vi "WaitBallTrajSkill.vi"(6 "passer tactic":T1=enum."PenaltyAttacker", 7 "firstCall":bool, 8 "error in (no error)":errorcluster, 9 "Robot":refnum<class "Robot.lvclass">, 10 "Game":refnum<class "Game.lvclass">, 11 "WaitBallTrajSkill in":refnum<class "WaitBallTrajSkill.lvclass">) -> (0 "error out":errorcluster, 2 "robot out":refnum<class "Robot.lvclass">, 3 "WaitBallTrajSkill out":refnum<class "WaitBallTrajSkill.lvclass">)   [LabVIEW 2024, in "WaitBallTrajSkill.lvclass"]
uses:
  WaitBallTrajSkill.lvclass
  Game_class/Game.lvclass
  Robot_class/Robot.lvclass
  C:/Users/moise/Documents/GitHub/SSL_AI/Object_class/Object.lvclass
  Robot_class/tactics.ctl
  Robot_class/robotKickToStates.ctl
  Robot_class/roles.ctl
  Robot_class/Robot.lvclass/Robot.ctl
  Object_class/Object.lvclass/Object.ctl
  Game_class/Game.lvclass/Game.ctl
  Parameters_class/Parameters.lvclass/Parameters.ctl
  Team_class/Team.lvclass/Team.ctl
  Ball_class/Ball.lvclass/Ball.ctl
  Field_class/Field.lvclass/Field.ctl
  Parameters_class/Read KickForce.vi
  Game_class/Read Parameters.lvclass.vi
  Game_class/Read BallRef.vi
  Game_class/Read Utilities.lvclass.vi
  Game_class/Read FieldRef.vi
  Game_class/Read NewParameters.vi
  Game_class/Read KeeperTeam.vi
  Game_class/Read OffensiveTeam.vi
  Team_class/Read RobotRef.vi
  Team_class/Read KeeperPlay.vi
  Field_class/Read ourGoalPosition.vi
  Field_class/Read enemyGoalPosition.vi
  Object_class/Read position(x,y).vi
  Ball_class/Read velocityNorm.vi
  Parameters_class/Read BallVelToAbortPass.vi
  Parameters_class/Read AttakingOurselves.vi
  Robot_class/Read Zone.vi
  Robot_class/Write robotKickState.vi
  Robot_class/Write dest_x.vi
  Robot_class/Write dest_y.vi
  Robot_class/Write dest_orientation.vi
  Robot_class/Write dribble.vi
  Robot_class/Write kick_x.vi
  Robot_class/Write keepDest.vi
  <vilib>/Analysis/_algsub.llb/Vector Norm.vi
  <vilib>/Analysis/_algsub.llb/Real Vector Norm.vi
  Ally_class/Ally.lvclass
  C:/Users/moise/Documents/GitHub/SSL_AI/Team_class/Team.lvclass
  Ball_class/Ball.lvclass
  Parameters_class/Parameters.lvclass
  Utilities_class/Utilities.lvclass
  Field_class/Field.lvclass
  Zone_class/Zone.lvclass
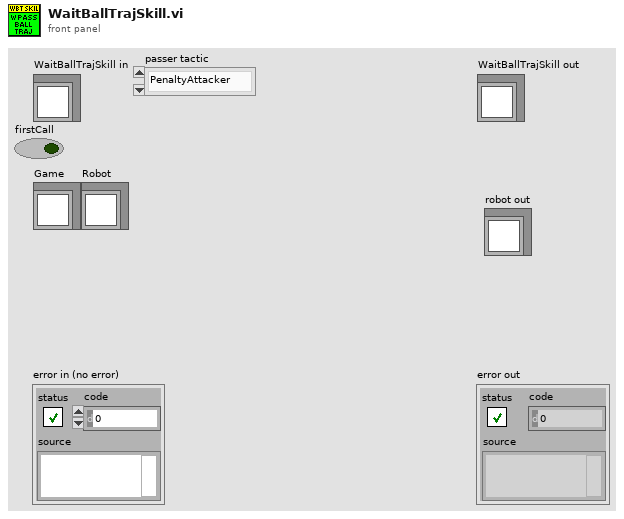
[diagram p1: front panel]
types:
  T1 = typedef "tactics.ctl" = enum16{"GoToBallPlacementPosition", "PlaceBall", "GoToBallPlacement", "5Robots", "BallPlacementEnemy", "ReceivePassInFuturePoint", "Roller", "PrepareRollToPassRollerGoTo", "PrepareRollToPassReceiverGoTo", "WaitRoll", "PositionToRoll", "PenaltyAttacker", "PassObserver", "PenaltyDefense", "TableReceiverTactic", "Test", "DefendGoal", "Marker", "FollowAttacker", "DefendArea", "Shoot", "AttackerAimGoal", "AttackerBallOutOfField", "AttackerBlock", "AttackerStop", "Duelist", "Halt", "ZigZag", "GoTo", "Timeout", "KickToBestRobot", "KickToPassReceiver", "PositionToReceivePass", "WaitPass", "GoToTarget"}
  T2 = typedef "robotKickToStates.ctl" = enum16{"shootFromDirect", "avoidCollideBall", "goToBackBall", "none", "walk", "turn", "turnAntiClockWise", "turnClockwise", "oldKickToShoot", "oldKickToGoToBackBall", "shoot"}
  T3 = typedef "roles.ctl" = enum16{"SimpleBallPlacement", "BallPlacementAllyPasser", "BallPlacementAllyReceiver", "BallPlacementEnemy", "5Robots5th", "PassBestReceiver", "5Robots4th", "5Robots3rd", "5Robots2nd", "5Robots1st", "PassBestRobot", "WaitPass", "ABCThirdKicker", "ABCFirstKicker", "ABCSecondKicker", "Tabler", "TableFinalizer", "PrepareRollToPassRoller", "PrepareRollToPassReceiver", "SimplePassRoll", "SimplePassRollReceiver", "PenaltyDefense", "PreparePassReceiver 2", "PreparePassReceiver 1", "PassObserver", "Timeout", "Goto", "ZigZag", "None", "BallOutOfField", "DefenderArea", "Duelist", "AttackerStop", "FollowAttacker", "KeeperRole", "KickPenalty", "AttackerAimGoal", "AttackerBlock", "Marker", "Halt", "Shoot", "PassKicker", "PassReceiver", "TestRole", "PenaltyAttacker"}
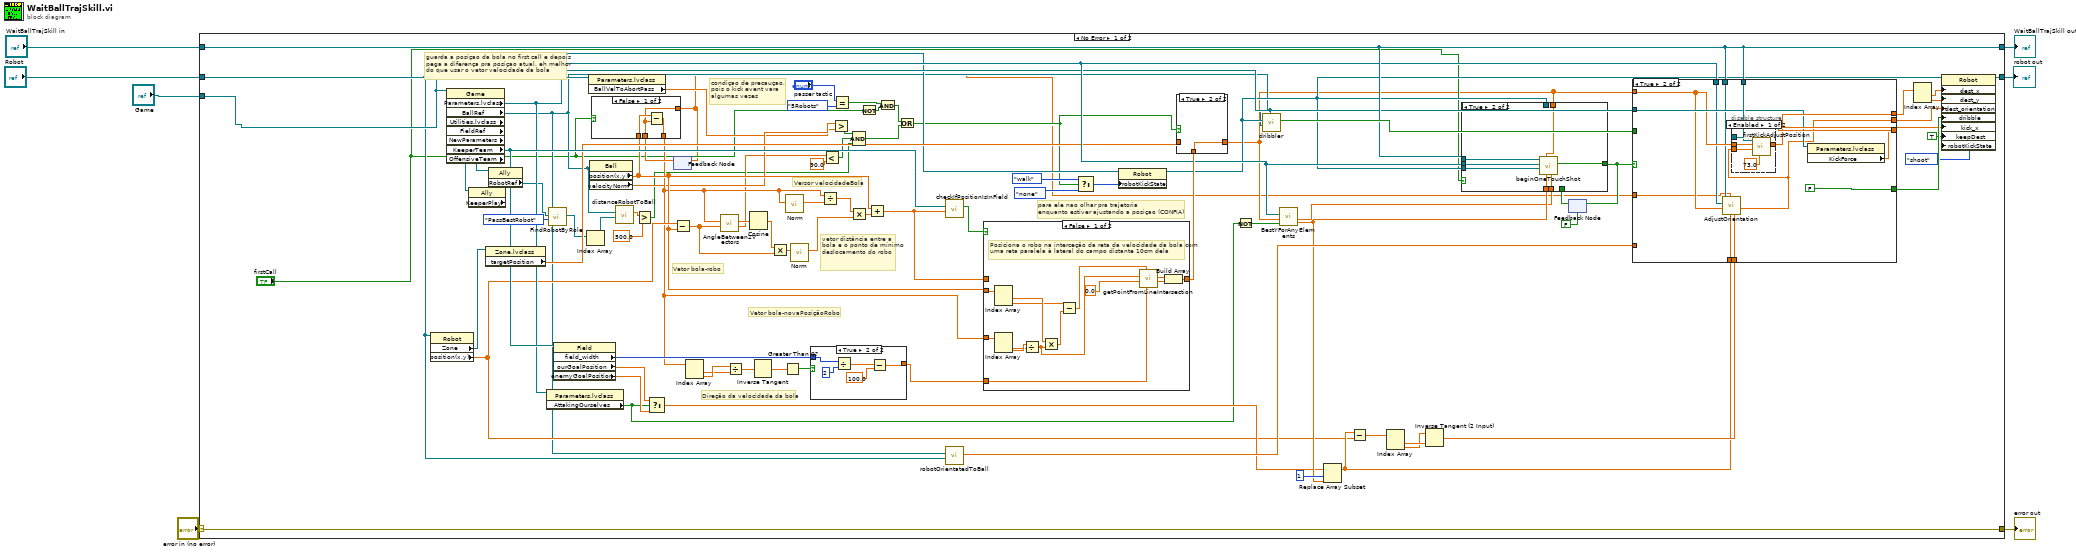
[diagram p0: block diagram]
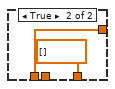
[diagram p2: hidden frame]
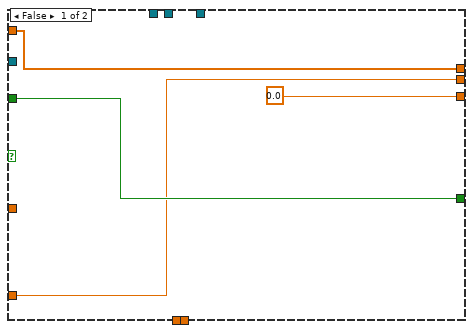
[diagram p4: hidden frame]
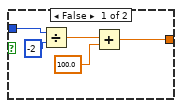
[diagram p7: hidden frame]
diagram:
  n1 = case shown="No Error" "error in (no error)" {
    selector: "error in (no error)" -> [w94 w158]
    tunnel: [w94 w158] -> w6
    tunnel: [w57 w157] -> w4
    tunnel: "WaitBallTrajSkill in" -> [w57 w157]
    tunnel: "Robot" -> [w42 _]
    tunnel: "Game" -> [w56 _]
    tunnel: [w93 _] -> w2
    frame No Error {
      # "guarda a posiçao da bola no first call e depois\npega a diferença pra posiçao atual. eh melhor\ndo que usar o vetor velocidade da bola"
      # "condiçao de precauçao,\npois o kick event vara \nalgumas vezes"
      # "para ele nao olhar pra trajetoria \nenquanto estiver ajustando a posiçao (CONFIA)"
      # "vetor distância entre a bola e o ponto de mínimo deslocamento do robo"
      # "Versor velocidadeBola"
      # "Direção da velocidade da bola"
      # "Vetor bola-novaPosiçãoRobo"
      # "Vetor bola-robo"
      n2 = property class="Robot"(reference=w42) -> ("Zone"=w45:refnum<class "Zone.lvclass">, "position(x,y)"=w46:dbl[])  [unwired: 1 in, 2 out]
      n3 = property class="Game" props=["Parameters.lvclass", "BallRef", "Utilities.lvclass", "FieldRef", "NewParameters", "KeeperTeam", "OffensiveTeam"](reference=w56) -> ("Parameters.lvclass"=w47:refnum<class "Parameters.lvclass">, "BallRef"=w15:refnum<class "Ball.lvclass">, "FieldRef"=w79:refnum<class "Field.lvclass">, "KeeperTeam"=w69:refnum<class "Ally.lvclass">, "OffensiveTeam"=w19:refnum<class "Ally.lvclass">)  [unwired: 1 in, 4 out]
      n4 = property class="Ally" props=["KeeperPlay"](reference=w69) -> ()  [unwired: 1 in, 3 out]
      n5 = property class="Zone.lvclass"(reference=w45) -> ("targetPosition"=w44:dbl[])  [unwired: 1 in, 2 out]
      n6 = property class="Ally"(reference=w19) -> ("RobotRef"=w18:refnum<class "Robot.lvclass">[])  [unwired: 1 in, 2 out]
      n7 = property class="Parameters.lvclass"(reference=w47) -> ("AttakingOurselves"=w51:bool)  [unwired: 1 in, 2 out]
      n8 = call "FindRobotByRole.vi"("role"=roles."PassBestRobot", "RobotRef"=w18) -> ("Robots"=w17:refnum<class "Robot.lvclass">[])  [unwired: 6 in, 3 out]
      n9 = property class="Field"(reference=w79) -> ("field_width"=w70:i32, "ourGoalPosition"=w54:dbl[], "enemyGoalPosition"=w53:dbl[])  [unwired: 1 in, 2 out]
      n10 = Index Array(array=w17) -> (element=w16:refnum<class "Robot.lvclass">)  [unwired: 1 in]
      n11 = property class="Parameters.lvclass"(reference=w47) -> ("BallVelToAbortPass"=w26:dbl)  [unwired: 1 in, 2 out]
      n12 = property class="Ball"(reference=w15) -> ("position(x,y)"=w33:dbl[], "velocityNorm"=w27:dbl)  [unwired: 1 in, 2 out]
      n13 = call "distanceRobotToBall.vi"("Robot"=w16, "Ball"=w15) -> ("Distance Robot To Ball"=w14:dbl)  [unwired: 7 in, 2 out]
      n14 = Greater?(x=w14, y=500.0) -> (0:w12:bool)
      n15 = Select(t=w54, s=w51, f=w53) -> (s? t:f=w52:dbl[])
      n16 = feedback #1() -> (w32:dbl[])  [unwired: 1 in]
      n17 = case shown="False" "firstCall" {
        tunnel: w33 -> [w97 w99]
        tunnel: w32 -> [w96 _]
        tunnel: [w96 w99] -> w9
        tunnel: [w95 dbl[] []] -> w30
        frame False {
          n18 = Subtract(x=w97, y=w96) -> (x-y=w95:dbl[])
        }
        frame True {
        }
      }
      n19 = feedback-in #1(w9) -> ()
      n20 = Subtract(x=w46, y=w33) -> (x-y=w43:dbl[])
      n21 = Index Array(array=w30) -> (element #1=w88:dbl, element #2=w89:dbl)  [unwired: 2 in]
      n22 = call "AngleBetween2Vectors.vi"("Array 1"=w43, "Array 2"=w30) -> ("angleInDegrees"=w21:dbl, "angleInRadians(default)"=w48:dbl)  [unwired: 6 in, 2 out]
      n23 = Divide(x=w89, y=w88) -> (x/y=w87:dbl)
      n24 = Cosine(x=w48) -> (cos(x)=w92:dbl)
      n25 = Inverse Tangent(1:w87) -> (0:w62:dbl)
      n26 = Multiply(x=w92, y=w43) -> (x*y=w83:dbl[])
      n27 = Greater Than 0?(x=w62) -> (x > 0?=w86:bool)
      n28 = call "Norm.vi"("2D vector"=w30) -> ("Modulo"=w31:dbl)  [unwired: 8 in, 2 out]
      n29 = call "Norm.vi"("2D vector"=w83) -> ("Modulo"=w80:dbl)  [unwired: 8 in, 2 out]
      n30 = case shown="True" w86 {
        tunnel: [w135 w140] -> w85
        tunnel: w70 -> [w132 w137]
        frame False {
          n31 = Divide(x=w132, y=-2) -> (x/y=w134:dbl)
          n32 = Add(x=w134, y=100.0) -> (x+y=w135:dbl)
        }
        frame True {
          n33 = Divide(x=w137, y=2) -> (x/y=w139:dbl)
          n34 = Subtract(x=w139, y=100.0) -> (x-y=w140:dbl)
        }
      }
      n35 = Divide(x=w30, y=w31) -> (x/y=w81:dbl[])
      n36 = Less?(x=w21, y=90.0) -> (x < y?=w23:bool)
      n37 = Greater?(x=w27, y=w26) -> (0:w25:bool)
      n38 = Equal?(x="passer tactic", y=tactics."5Robots") -> (x = y?=w35:bool)
      n39 = Multiply(x=w81, y=w80) -> (x*y=w82:dbl[])
      n40 = Compound Arithmetic op=AND(w25, w23, w12) -> (w24:bool)
      n41 = Not(x="firstCall") -> (.not. x?=w34:bool)
      n42 = Add(x=w33, y=w82) -> (x+y=w90:dbl[])
      n43 = And(x=w35, y=w34) -> (x .and. y?=w29:bool)
      n44 = Or(x=w29, y=w24) -> (x .or. y?=w28:bool)
      n45 = call "checkIfPositionIsInField.vi"("Position"=w90, "FieldRef"=w79) -> ("Position Is In Field?"=w91:bool)  [unwired: 5 in, 4 out]
      n46 = call "robotOrientatedToBall.vi"("Robot"=w42, "BallRef"=w15) -> ("Orientation"=w74:dbl)  [unwired: 7 in, 2 out]
      n47 = case shown="False" w91 {
        tunnel: w90 -> [_ w156]
        tunnel: [w153 w156] -> w84
        tunnel: w85 -> [w151 _]
        tunnel: w33 -> [w150 _]
        tunnel: w30 -> [w149 _]
        frame False {
          # "Posiciona o robo na interceção da reta da velocidade da bola com uma reta paralela à lateral do campo distante 10cm dela"
          n48 = Index Array(array=w149) -> (element #1=w147:dbl, element #2=w148:dbl)  [unwired: 2 in]
          n49 = Index Array(array=w150) -> (element #1=w146:dbl, element #2=w145:dbl)  [unwired: 2 in]
          n50 = Divide(x=w148, y=w147) -> (x/y=w142:dbl)
          n51 = Multiply(x=w146, y=w142) -> (x*y=w144:dbl)
          n52 = Subtract(x=w145, y=w144) -> (x-y=w143:dbl)
          n53 = call "getPointFromLineIntersection.vi"("b2"=w151, "b1"=w143, "a2"=0.0, "a1"=w142) -> ("y_intersection"=w154:dbl, "x_intersection"=w155:dbl)  [unwired: 4 in, 2 out]
          n54 = Build Array(w155, w154) -> (w153:dbl[])
        }
        frame True {
        }
      }
      n55 = Select(t=robotKickToStates."walk" ("robotKickState"), s=w28, f=robotKickToStates."none" ("robotKickState")) -> (s? t:f=w38:T2)
      n56 = property class="Robot"(reference=w42, "robotKickState"=w38) -> (reference out=w41:refnum<class "Robot.lvclass">)  [unwired: 1 in, 1 out]
      n57 = case shown="True" w28 {
        tunnel: w84 -> [_ w131]
        tunnel: [w130 w131] -> w10
        tunnel: w44 -> [w130 _]
        frame False {
        }
        frame True {
        }
      }
      n58 = Not(x=w51) -> (.not. x?=w50:bool)
      n59 = call "dribbler.vi"("Parameters.lvclass"=w47, "Ball"=w15, "Robot"=w41) -> ("Dribbler?"=w77:bool)  [unwired: 6 in, 2 out]
      n60 = call "BestYForAnyElements.vi"("inimigos"=w50, "Position to be analyzed"=w10, "Game"=w56) -> ("Best y"=w55:dbl, "Gap Coord"=w49:dbl[])  [unwired: 5 in, 2 out]
      n61 = Replace Array Subset(array=w52, new element=w55, index=1) -> (w58:dbl[])
      n62 = Subtract(x=w58, y=w46) -> (x-y=w71:dbl[])
      n63 = Index Array(array=w71) -> (element #1=w73:dbl, element #2=w72:dbl)  [unwired: 2 in]
      n64 = Inverse Tangent (2 Input)(1:w73, 2:w72) -> (0:w59:dbl)
      n65 = feedback #2(FALSE ("Boolean")) -> (w64:bool)
      n66 = case shown="True" "firstCall" {
        tunnel: w57 -> [_ w107]
        tunnel: w56 -> [_ w106]
        tunnel: w41 -> [_ w105]
        tunnel: [w100 w104] -> w65
        tunnel: w64 -> [w100 _]
        tunnel: w41 -> [_ _]
        tunnel: w55 -> [_ w103]
        tunnel: w49 -> [_ w102]
        tunnel: w10 -> [_ w101]
        frame False {
        }
        frame True {
          n67 = call "beginOneTouchShot.vi"("Gap Coord"=w102, "bestY"=w103, "targetPosition"=w101, "Robot"=w105, "Game"=w106, "WaitBallTrajSkill in"=w107) -> ("Boolean"=w104:bool)  [unwired: 3 in, 2 out]
        }
      }
      n68 = feedback-in #2(w65) -> ()
      n69 = case shown="True" w65 {
        tunnel: [w111 FALSE ("Dribbler?")] -> w78
        tunnel: w77 -> [w111 _]
        tunnel: [w110 w113] -> w76
        tunnel: w74 -> [w110 _]
        tunnel: [0.0 ("kick_x") w119] -> w75
        tunnel: w47 -> [_ w120]
        tunnel: w57 -> [_ w122]
        tunnel: w10 -> [w108 w116]
        tunnel: [w108 w121] -> w68
        tunnel: w59 -> [_ w118]
        tunnel: w58 -> [_ w117]
        tunnel: w56 -> [_ w115]
        tunnel: w57 -> [_ w114]
        tunnel: w9 -> [_ w112]
        frame False {
        }
        frame True {
          n70 = call "AdjustOrientation.vi"("orientation"=w118, "target"=w117, "initial pos"=w112, "dest"=w116, "Game"=w115, "WaitBallTrajSkill in"=w114) -> ("orientation out"=w113:dbl)  [unwired: 3 in, 2 out]
          n71 = disable-structure shown="Enabled" {
            disable-tunnel: w122 -> [w128 _]
            disable-tunnel: [w127 w129] -> w121
            disable-tunnel: w116 -> [w125 w129]
            disable-tunnel: w113 -> [w124 _]
            frame Enabled {
              n72 = call "firstKickAdjustPosition.vi"("Dist"=73.0, "Orientation"=w124, "Dest"=w125, "WaitBallTrajSkill in"=w128) -> ("AdjustDest"=w127:dbl[])  [unwired: 5 in, 2 out]
            }
            frame Disabled {
            }
          }
          n73 = property class="Parameters.lvclass"(reference=w120) -> ("KickForce"=w119:dbl)  [unwired: 1 in, 2 out]
        }
      }
      n74 = Index Array(array=w68) -> (element #1=w66:dbl, element #2=w67:dbl)  [unwired: 2 in]
      n75 = property class="Robot"(reference=w41, "dest_x"=w66, "dest_y"=w67, "dest_orientation"=w76, "dribble"=w78, "kick_x"=w75, "keepDest"=TRUE, "robotKickState"=robotKickToStates."shoot") -> (reference out=w93:refnum<class "Robot.lvclass">)  [unwired: 1 in, 1 out]
    }
    frame Error {
    }
  }
  "error out" <- w6
  "WaitBallTrajSkill out" <- w4
  "robot out" <- w2
